vi "Digital IO Message - Continuous Port Report.vi"(8 "error in (no error)":errorcluster, 9 "Enable Continuous Reporting?":bool, 10 "Port Index":u8 format="%x", 11 "Refnum In":refnum<vi>) -> (0 "error out":errorcluster, 1 "PortValue":u16, 2 "Port Index Out":u8, 3 "Refnum Out":refnum<vi>, 4 "PortValueAsArray":bool[](array[boolean]))   [LabVIEW 2020]
doc: "Allows requesting the state of a digital port."
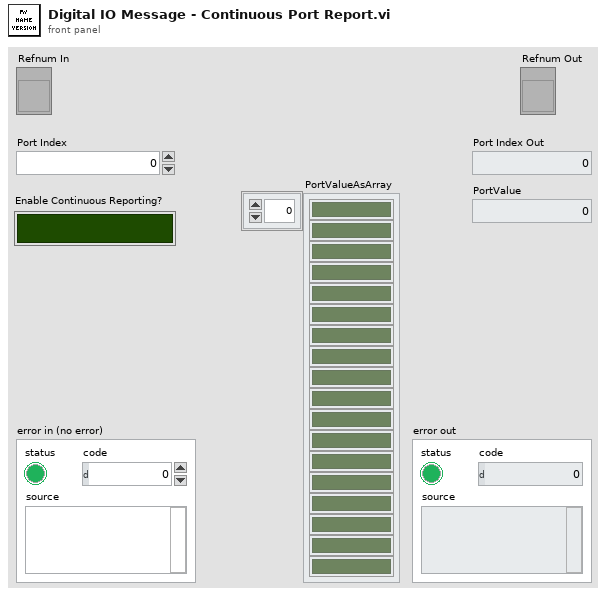
[diagram p1: front panel]
types:
  T1 = typedef "FirmataProtocolConstants.ctl" = u16
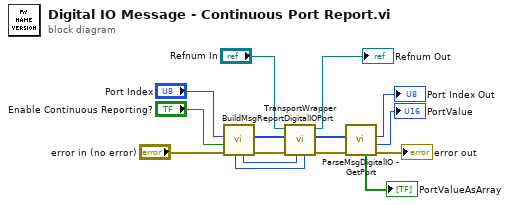
[diagram p0: block diagram]
diagram:
  n1 = call "BuildMsgReportDigitalIOPort.vi"("error in"="error in (no error)", "Enable Continuous Reporting?"="Enable Continuous Reporting?", "Port Index"="Port Index") -> ("error out"=w15:errorcluster, "DigitalIOMessage"=w9:u8[], "ReplyFirstByte"=w10:T1, "ReplyLength"=w11:i32)  [unwired: 5 in]
  n2 = call "TransportWrapper.vi"("ReplyLength"=w11, "ReplyFirstByte"=w10, "error in"=w15, "Message In"=w9, "Refnum In"="Refnum In") -> ("error out"=w6:errorcluster, "Message Out"=w4:u8[], "Refnum Out"=→"Refnum Out":refnum<vi>)  [unwired: 4 in]
  n3 = call "ParseMsgDigitalIO - GetPort.vi"("error in"=w6, "Message"=w4) -> ("error out"=→"error out":errorcluster, "PortValue"=→"PortValue":u16, "Port Index"=→"Port Index Out":u8, "PortValueAsArray"=→"PortValueAsArray":bool[])  [unwired: 6 in]
